vi "visitRectangle.vi"(8 "error in (no error)":errorcluster, 10 "Rectangle":refnum<class "Rectangle.lvclass">, 11 "Visitor in":refnum<class "Visitor.lvclass">) -> (0 "error out":errorcluster, 2 "String":string, 3 "Visitor out":refnum<class "Visitor.lvclass">)   [LabVIEW 2017, in "Visitor.lvclass"]
uses:
  Visitor.lvclass
  Rectangle Class/Rectangle.lvclass
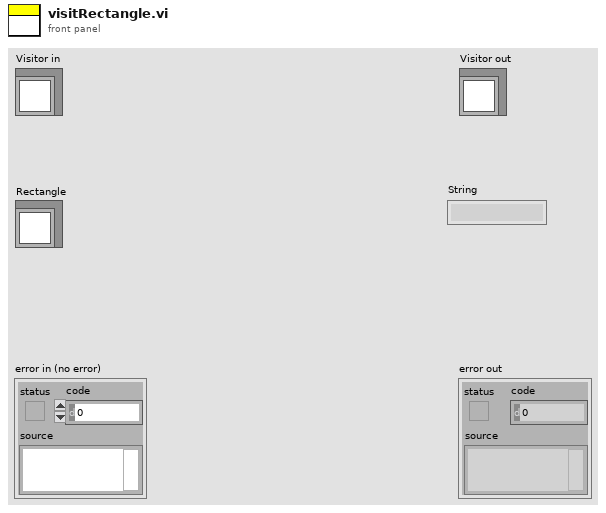
[diagram p1: front panel]
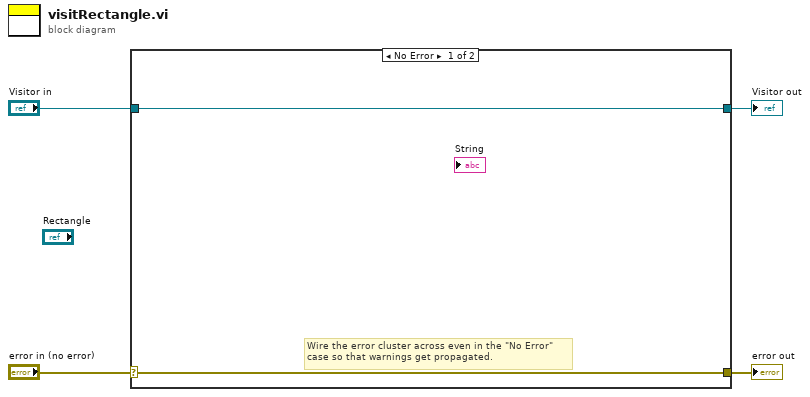
[diagram p0: block diagram]
diagram:
  n1 = case shown="No Error" "error in (no error)" {
    selector: "error in (no error)" -> [w5 w8]
    tunnel: [w5 w8] -> w3
    tunnel: [w6 w7] -> w1
    tunnel: "Visitor in" -> [w6 w7]
    frame No Error {
      # "Wire the error cluster across even in the \"No Error\"\ncase so that warnings get propagated."
    }
    frame Error {
    }
  }
  "error out" <- w3
  "Visitor out" <- w1
